vi "Data Logger.vi"(6 "PN In":string, 7 "Test Result?":bool, 8 "Error In":errorcluster, 9 "DB File":path=path "D:/dB/testdata.s3db", 10 "Model (F-ME74)":bool, 11 "Test Data In":string[](array[string])) -> (0 "Error Out":errorcluster, 1 "LBL Data":T1, 2 "Full SN":string)   [LabVIEW 2018]
uses:
  <vilib>/drjdpowell/SQLite Library/SQL Connection/Connection.lvclass/Connection.ctl
  <vilib>/drjdpowell/SQLite Library/SQL Connection/Open (path).vi
  <vilib>/drjdpowell/SQLite Library/SQL Connection/Open (string).vi
  <vilib>/AdvancedString/Path To Command Line String.vi
  <vilib>/drjdpowell/SQLite Library/SQL Connection/Execute SQL (1D String).vi
  <vilib>/drjdpowell/SQLite Library/SQL Connection/Execute SQL (Single Integer).vi
  <vilib>/drjdpowell/SQLite Library/SQL Connection/Connection.lvclass
  <vilib>/drjdpowell/SQLite Library/SQLite.lvlib
panel:
  out "Last MFG DT":string
  out "Insert SQL":string
  # "Test Data Logger to Data Base"
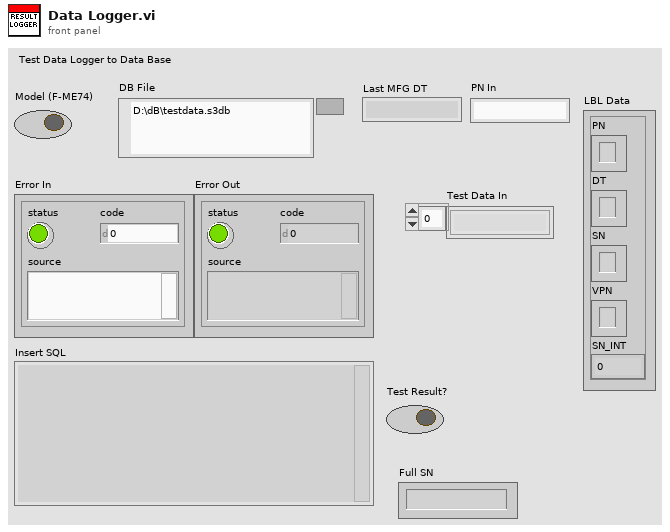
[diagram p1: front panel]
types:
  T1 = cluster{"PN":string, "DT":string, "SN":string, "VPN":string, "SN_INT":i32}
  T2 = enum16{"New or existing", "Existing", "Read only"}
  T3 = cluster{"PN In":string, "DATE And SHIFT":string, "SN":string, string, "Last INSERT RowID":i64}
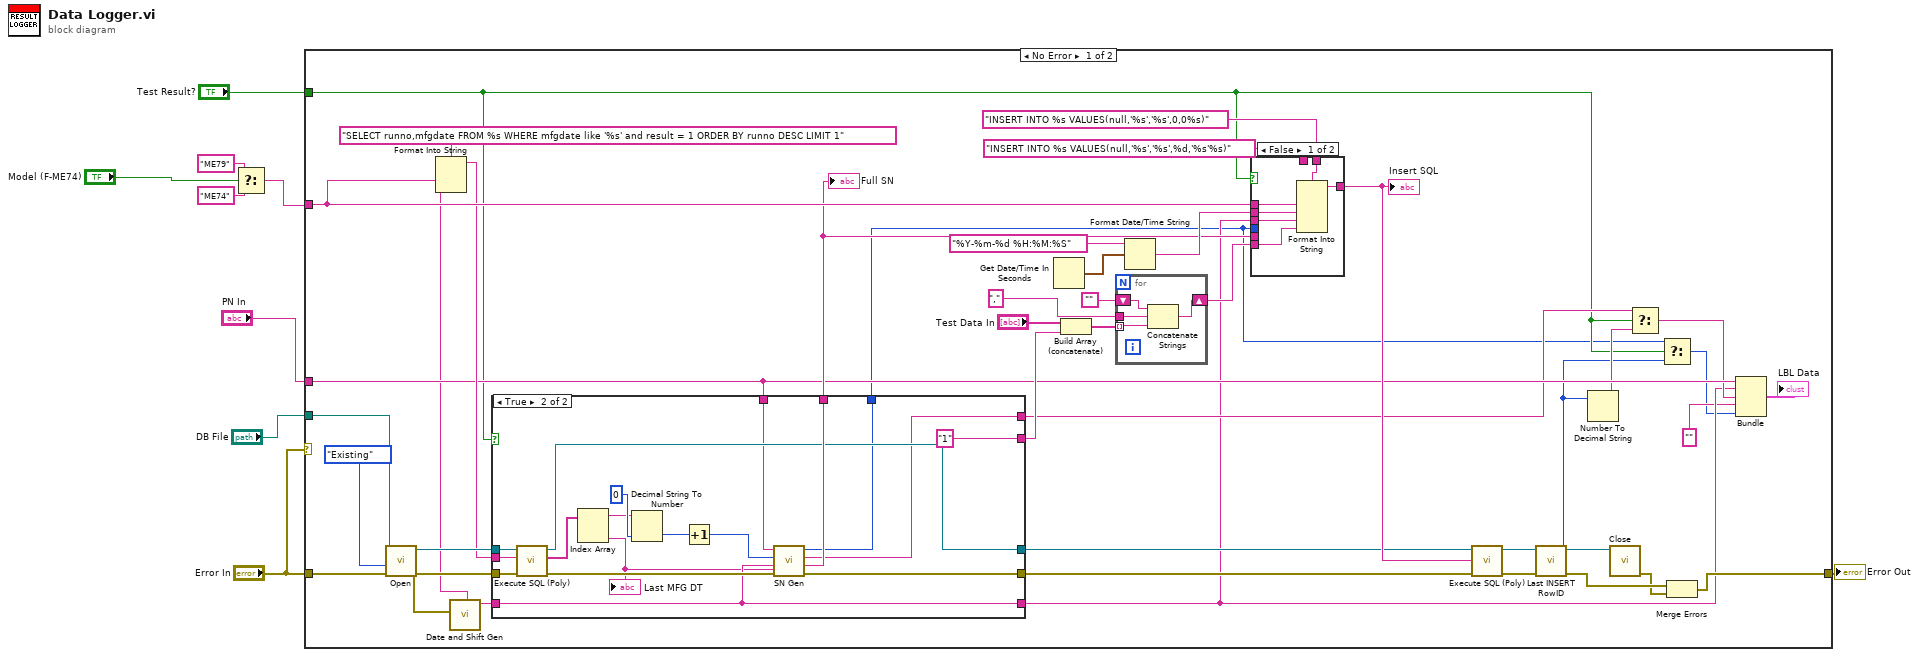
[diagram p0: block diagram]
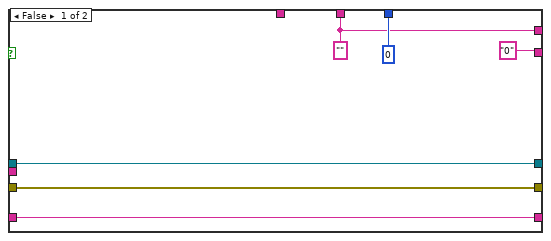
[diagram p2: hidden frame]
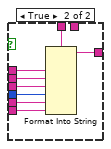
[diagram p3: hidden frame]
diagram:
  n1 = Select(t="ME79", s="Model (F-ME74)", f="ME74") -> (s? t:f=w4:string)
  n2 = case shown="No Error" "Error In" {
    tunnel: "Error In" -> [w50 w94]
    tunnel: "DB File" -> [w49 _]
    tunnel: [w24 w94] -> w7
    tunnel: w4 -> [w41 _]
    tunnel: "PN In" -> [w20 _]
    tunnel: "Test Result?" -> [w13 _]
    frame No Error {
      n3 = call-poly <vilib>:"Open.vi"("error in (no error)"=w50, "File Option"=T2."Existing", "db file"=w49) -> ("error out"=w23:errorcluster, "SQLite Connection"=w40:refnum<class "Connection.lvclass">)  [unwired: 7 in]
      n4 = call "Date and Shift Gen.vi"("Error In"=w23) -> ("DATE And SHIFT"=w22:string, "MFG Date for SQL"=w15:string)  [unwired: 8 in, 1 out]
      n5 = Format Into String(format string="SELECT runno,mfgdate FROM %s WHERE mfgdate like '%s' and result = 1 ORDER BY runno DESC LIMIT 1", w41, w15) -> (resulting string=w39:string)  [unwired: 2 in, 1 out]
      n6 = case shown="True" w13 {
        tunnel: w23 -> [w57 w75]
        tunnel: w40 -> [w56 w74]
        tunnel: w39 -> [_ w73]
        tunnel: w20 -> [_ w68]
        tunnel: [i64 0 w58] -> w12
        tunnel: [w53 w72] -> w33
        tunnel: [w57 w71] -> w36
        tunnel: [w56 w70] -> w35
        tunnel: ["0" "1"] -> w30
        tunnel: [w53 w67] -> w19
        tunnel: w22 -> [w52 w65]
        tunnel: [w52 w65] -> w16
        frame False {
          w53 = "" ("SN Out")
        }
        frame True {
          n7 = call-poly <vilib>:"Execute SQL (Poly).vi"("error in (no error)"=w75, "SQL"=w73, "SQLite Connection in"=w74) -> ("error out"=w66:errorcluster, "Result Set"=w64:string[], "SQLite Connection"=w70:refnum<class "Connection.lvclass">)  [unwired: 5 in, 1 out]
          n8 = Index Array(array=w64) -> (element #1=w62:string, element #2=w59:string)  [unwired: 2 in]
          "Last MFG DT" <- w59
          n9 = Decimal String To Number(string=w62, default (0L)=0 ("default (0 I32)")) -> (number=w61:i32)  [unwired: 1 in, 1 out]
          n10 = Increment(x=w61) -> (x+1=w60:i32)
          n11 = call "SN Gen.vi"("Last MFG Date"=w59, "error in (no error)"=w66, "Date and Shift In"=w65, "SN In"=w60, "PN In"=w68) -> ("error out"=w71:errorcluster, "Full SN Out"=w72:string, "SN"=w67:string, "SN Out"=w58:i64)  [unwired: 3 in]
        }
      }
      "Full SN" <- w33
      n12 = Get Date/Time In Seconds() -> (seconds since 1Jan1904=w44:timestamp)
      n13 = Build Array (concatenate)("Test Data In", w30) -> (w47:string[])
      n14 = for {
        tunnel: w47 -> [w93] mode=indexing
        shift-right: [w90] -> w38
        shift-left: "" -> [w91]
        tunnel: "," -> [w92]
        n15 = Concatenate Strings(w91, w92, w93) -> (w90:string)
      }
      n16 = Format Date/Time String(time format string (%c)="%Y-%m-%d %H:%M:%S", seconds (now)=w44) -> (date/time string=w37:string)  [unwired: 1 in]
      n17 = case shown="False" w13 {
        tunnel: "INSERT INTO %s VALUES(null,'%s','%s',%d,'%s'%s)" -> [_ w89]
        tunnel: [w79 w88] -> w45
        tunnel: w41 -> [w80 w87]
        tunnel: w38 -> [w77 w86]
        tunnel: w37 -> [w78 w83]
        tunnel: "INSERT INTO %s VALUES(null,'%s','%s',0,0%s)" -> [w81 _]
        tunnel: w12 -> [_ w85]
        tunnel: w33 -> [_ w84]
        tunnel: w16 -> [w76 w82]
        frame False {
          n18 = Format Into String(format string=w81, w80, w78, w76, w77) -> (resulting string=w79:string)  [unwired: 2 in, 1 out]
        }
        frame True {
          n19 = Format Into String(format string=w89, w87, w83, w82, w85, w84, w86) -> (resulting string=w88:string)  [unwired: 2 in, 1 out]
        }
      }
      "Insert SQL" <- w45
      n20 = call-poly <vilib>:"Execute SQL (Poly).vi"("error in (no error)"=w36, "SQL"=w45, "SQLite Connection in"=w35) -> ("error out"=w29:errorcluster, "SQLite Connection"=w28:refnum<class "Connection.lvclass">)  [unwired: 6 in, 1 out]
      n21 = call <vilib>:"Last INSERT RowID.vi"("error in (no error)"=w29, "SQLite Connection in"=w28) -> ("error out"=w26:errorcluster, "Last INSERT RowID"=w11:i64, "SQLite Connection"=w27:refnum<class "Connection.lvclass">)  [unwired: 7 in]
      n22 = Number To Decimal String(number=w11) -> (decimal integer string=w18:string)  [unwired: 1 in]
      n23 = call-dynamic "Close.vi"("SQLite Connection in"=w27) -> ("error out"=w25:errorcluster)  [unwired: 10 in]
      n24 = Select(t=w19, s=w13, f=w18) -> (s? t:f=w17:string)
      n25 = Select(t=w12, s=w13, f=w11) -> (s? t:f=w10:i64)
      n26 = Merge Errors(w26, w25) -> (w24:errorcluster)
      n27 = Bundle("PN In"=w20, "DATE And SHIFT"=w16, "SN"=w17, "", "Last INSERT RowID"=w10) -> (→"LBL Data":T3)  [unwired: 1 in]
    }
    frame Error {
    }
  }
  "Error Out" <- w7
